vi "Control Type to String.vi"(7 "Term (Methods)":string="Methods", 10 "Lib Name":string, 11 "Control VI Type":T1(ring)) -> (3 "String":string)   [LabVIEW 2023, in "VIDoc Printer.lvlib" / "VIDoc Printer.lvclass"]
doc: "Converts the Control VI Type into a printable String."
uses:
  VIDoc Printer.lvclass
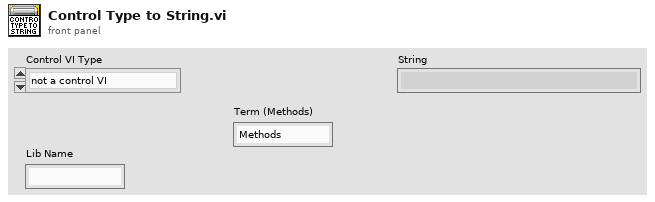
[diagram p1: front panel]
types:
  T1 = enum32{"not a control VI", "control", "typedef", "strict typedef"}
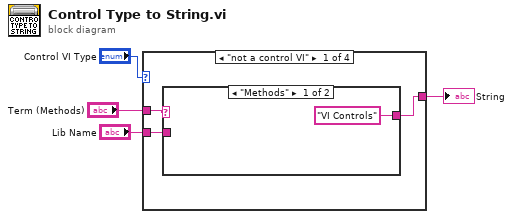
[diagram p0: block diagram]
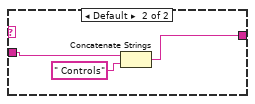
[diagram p2: hidden frame]
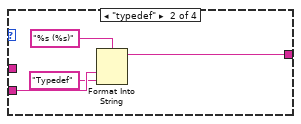
[diagram p3: hidden frame]
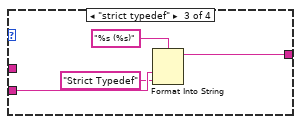
[diagram p4: hidden frame]
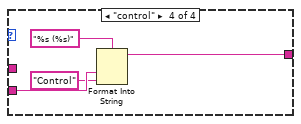
[diagram p5: hidden frame]
diagram:
  n1 = case shown="\"not a control VI\"" "Control VI Type" {
    tunnel: [w7 w13 w16 w20] -> w3
    tunnel: "Lib Name" -> [w6 w15 w18 w22]
    tunnel: "Term (Methods)" -> [w5 _ _ _]
    frame "not a control VI" {
      n2 = case shown="\"Methods\"" w5 {
        tunnel: ["VI Controls" w9] -> w7
        tunnel: w6 -> [_ w11]
        frame "Methods" {
        }
        frame Default {
          n3 = Concatenate Strings(w11, " Controls") -> (w9:string)
        }
      }
    }
    frame "typedef" {
      n4 = Format Into String(format string="%s (%s)", w15, "Typedef") -> (resulting string=w13:string)  [unwired: 2 in, 1 out]
    }
    frame "strict typedef" {
      n5 = Format Into String(format string="%s (%s)", w18, "Strict Typedef") -> (resulting string=w16:string)  [unwired: 2 in, 1 out]
    }
    frame "control" {
      n6 = Format Into String(format string="%s (%s)", w22, "Control") -> (resulting string=w20:string)  [unwired: 2 in, 1 out]
    }
  }
  "String" <- w3
